vi "prova.vi"() -> ()   [LabVIEW 2011]
uses:
  <vilib>/measure/mamon.llb/Waveform Peak Detection for 1 Chan.vi
  <vilib>/express/express analysis/Spectral/Block/exnSpectralBlock spectral measurements peak poly.vi
  <vilib>/express/express analysis/Spectral/Block/exnSpectralBlock spectral measurements peak DDT.vi
  <vilib>/express/express analysis/Spectral/XNode/ExpressSpectralMeasurementsBlockNode.xnode
  <vilib>/measure/NI_MAPro.lvlib
panel:
  out "Amplitudes":dbl[](array[numeric]) format="%.2p"
  out "Locations":dbl[](array[numeric]) format="%.2p"
  out "Filtered Signal 3":dynamicdata(graph) caption="Filtered Signal"
  in  "Lower Cut-Off":dbl=0.0001
  in  "Upper Cut-Off":dbl=0.005
  in  "stop":bool
  in  "dimension 0,003":i32=2000
  in  "dimension 0,002":i32=1000
  in  "dimension 0,01":i32=1000
  out "size(s)":i32
  out "Filtered Signal 2":dbl[](graph) caption="Filtered Signal"
  out "Filtered Signal":dynamicdata(graph)
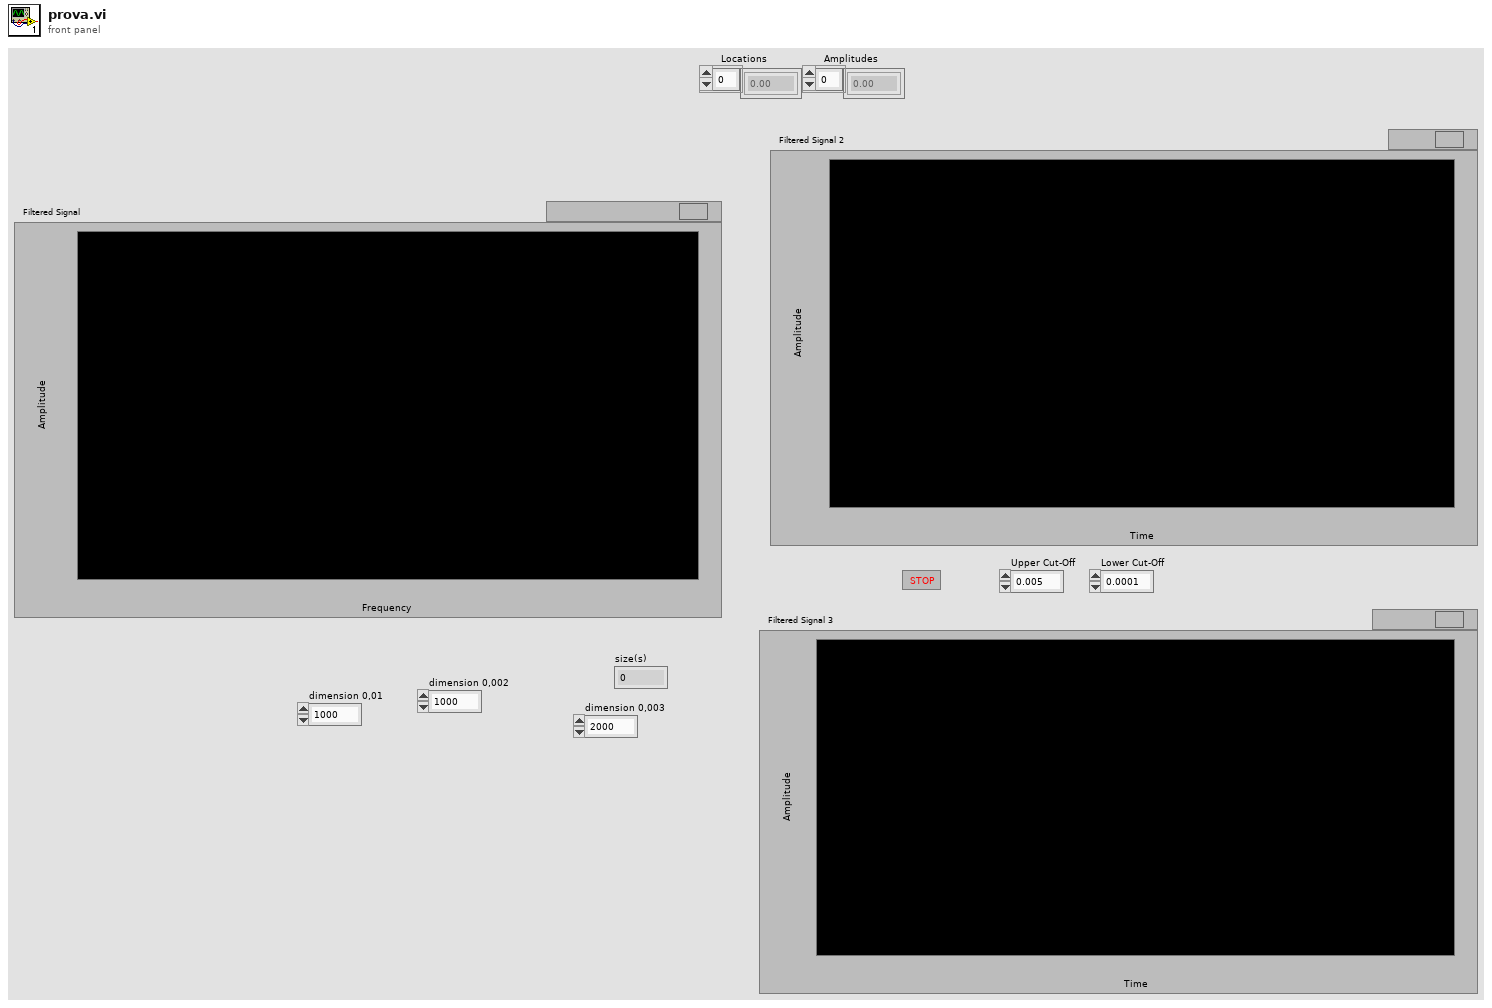
[diagram p1: front panel]
types:
  T1 = cluster{"averaging mode":u16, "weighting mode":u16, "number of averages":u32}
  T2 = cluster{"dB On (F)":bool, "unwrap phase (F)":bool, "convert to degree (F)":bool}
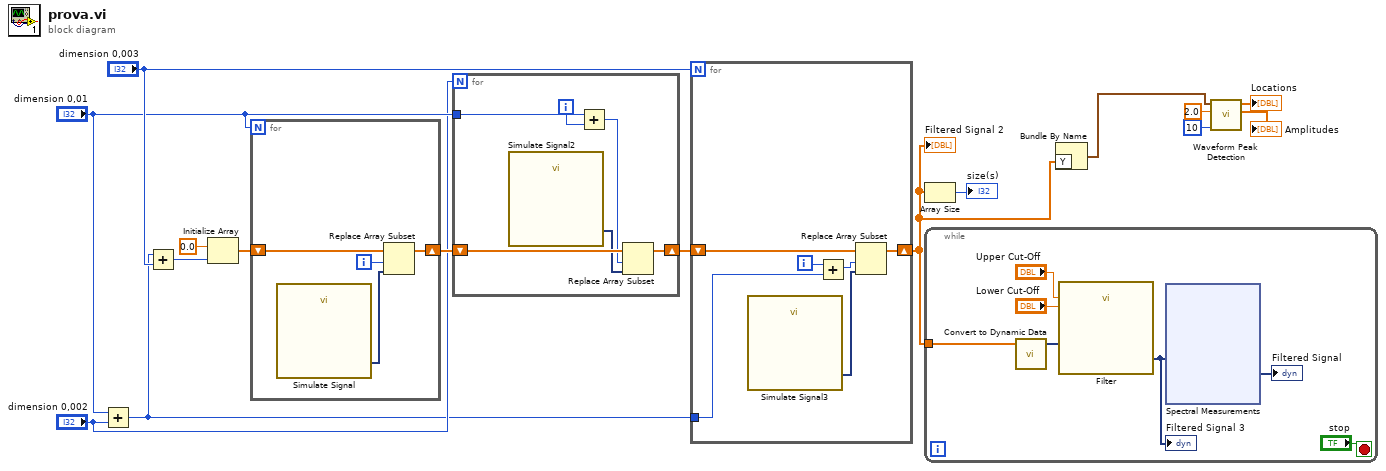
[diagram p0: block diagram]
diagram:
  n1 = Add(x="dimension 0,01", y="dimension 0,002") -> (x+y=w8:i32)
  n2 = Add(x=w8, y="dimension 0,003") -> (x+y=w12:i32)
  n3 = Initialize Array(0.0 ("element"), w12) -> (w16:dbl[])
  n4 = for {
    N: "dimension 0,01" -> [_]
    shift-right: [w17] -> w14
    shift-left: w16 -> [w20]
    i -> [w18]
    n5 = call "Simulate Signal"() -> ("Sine"=w19:dynamicdata)  [unwired: 14 in, 1 out]
    n6 = Replace Array Subset(array=w20, new element=w19, index=w18) -> (w17:dbl[])
  }
  n7 = for {
    N: "dimension 0,002" -> [_]
    shift-right: [w23] -> w13
    shift-left: w14 -> [w26]
    tunnel: "dimension 0,01" -> [w21]
    i -> [w24]
    n8 = call "Simulate Signal2"() -> ("Sine"=w25:dynamicdata)  [unwired: 14 in, 1 out]
    n9 = Add(x=w21, y=w24) -> (x+y=w22:i32)
    n10 = Replace Array Subset(array=w26, new element=w25, index=w22) -> (w23:dbl[])
  }
  n11 = for {
    N: "dimension 0,003" -> [_]
    shift-right: [w29] -> w5
    shift-left: w13 -> [w32]
    tunnel: w8 -> [w27]
    i -> [w30]
    n12 = call "Simulate Signal3"() -> ("Sine"=w31:dynamicdata)  [unwired: 14 in, 1 out]
    n13 = Add(x=w30, y=w27) -> (x+y=w28:i32)
    n14 = Replace Array Subset(array=w32, new element=w31, index=w28) -> (w29:dbl[])
  }
  "Filtered Signal 2" <- w5
  n15 = Array Size(array=w5) -> (size(s)=→"size(s)":i32)
  n16 = while {
    tunnel: w5 -> [w37]
    stop <- "stop" stop-if-true
    n17 = call "Convert to Dynamic Data"("Array"=w37) -> ("Dynamic Data Type"=w36:dynamicdata)  [unwired: 3 in]
    n18 = call "Filter"("Lower Cut-Off"="Lower Cut-Off", "Upper Cut-Off"="Upper Cut-Off", "Signal"=w36) -> ("Filtered Signal"=w35:dynamicdata)  [unwired: 7 in, 1 out]
    "Filtered Signal 3" <- w35
    n19 = xnode "Spectral Measurements"("Signals"=w35) -> ("FFT - (Peak)"=→"Filtered Signal":dynamicdata)  [unwired: 1 in, 2 out]
  }
  n20 = Bundle By Name("Y"=w5) -> (w4:waveform(dbl))  [unwired: 1 in]
  n21 = call-poly <vilib>:"Waveform Peak Detection.vi"("width"=10, "threshold"=2.0, "Signal In"=w4) -> ("Amplitudes"=→"Amplitudes":dbl[], "Locations"=→"Locations":dbl[])  [unwired: 4 in, 3 out]
